vi "Start_Hexap(sous-VI).vi"(10 "Login Credentials":T2={"Username"="root", "Password"="edison"}, 11 "Server Settings":T1={"Server IP Address"="192.168.43.226", "Server Port"=22}) -> ()   [LabVIEW 2019]
uses:
  <vilib>/Alab Technologies/ALAB SSH/Controls/Login Credentials.ctl
  <vilib>/Alab Technologies/ALAB SSH/Controls/Server Settings.ctl
  <vilib>/Alab Technologies/ALAB SSH/ALAB-SSH.lvlib
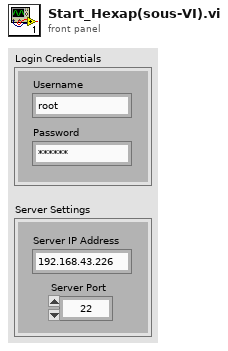
[diagram p1: front panel]
types:
  T1 = typedef "ALAB-SSH.lvlib/Server Settings.ctl" = cluster{"Server IP Address":string, "Server Port":i32}
  T2 = typedef "ALAB-SSH.lvlib/Login Credentials.ctl" = cluster{"Username":string, "Password":string}
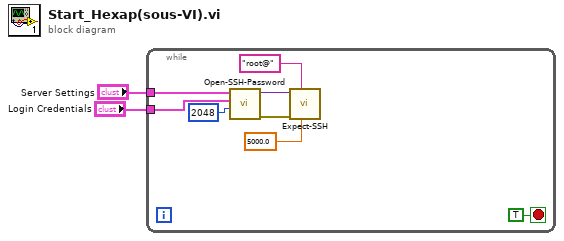
[diagram p0: block diagram]
diagram:
  n1 = while {
    tunnel: "Login Credentials" -> [w9]
    tunnel: "Server Settings" -> [w8]
    stop <- TRUE stop-if-true
    n2 = call <vilib>:"Open-SSH-Password.vi"("Buffer Size"=2048, "Login Credentials"=w9, "Server Settings"=w8) -> ("Error out"=w5:errorcluster, "SSH Session"=w6:variant)  [unwired: 7 in]
    n3 = call <vilib>:"Expect-SSH.vi"("Timeout (ms)"=5000.0, "Regular Expression"="root@", "Error in"=w5, "Session-In"=w6) -> ()  [unwired: 5 in, 3 out]
  }
